vi "only_x_and_y_output.vi"(11 "range":dbl) -> (0 "cycle 2":bool, 1 "range 2":dbl, 2 "Output Y":dbl, 3 "Output X":dbl)   [LabVIEW 2014]
panel:
  out "cycle":bool
  in  "GPIB In":refnum<visa-resource-name>="GPIB0::8::INSTR"
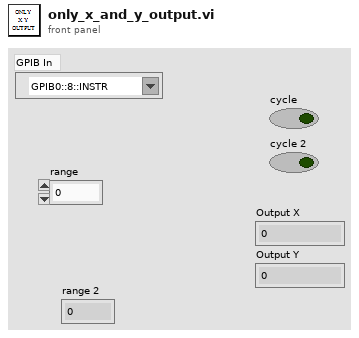
[diagram p1: front panel]
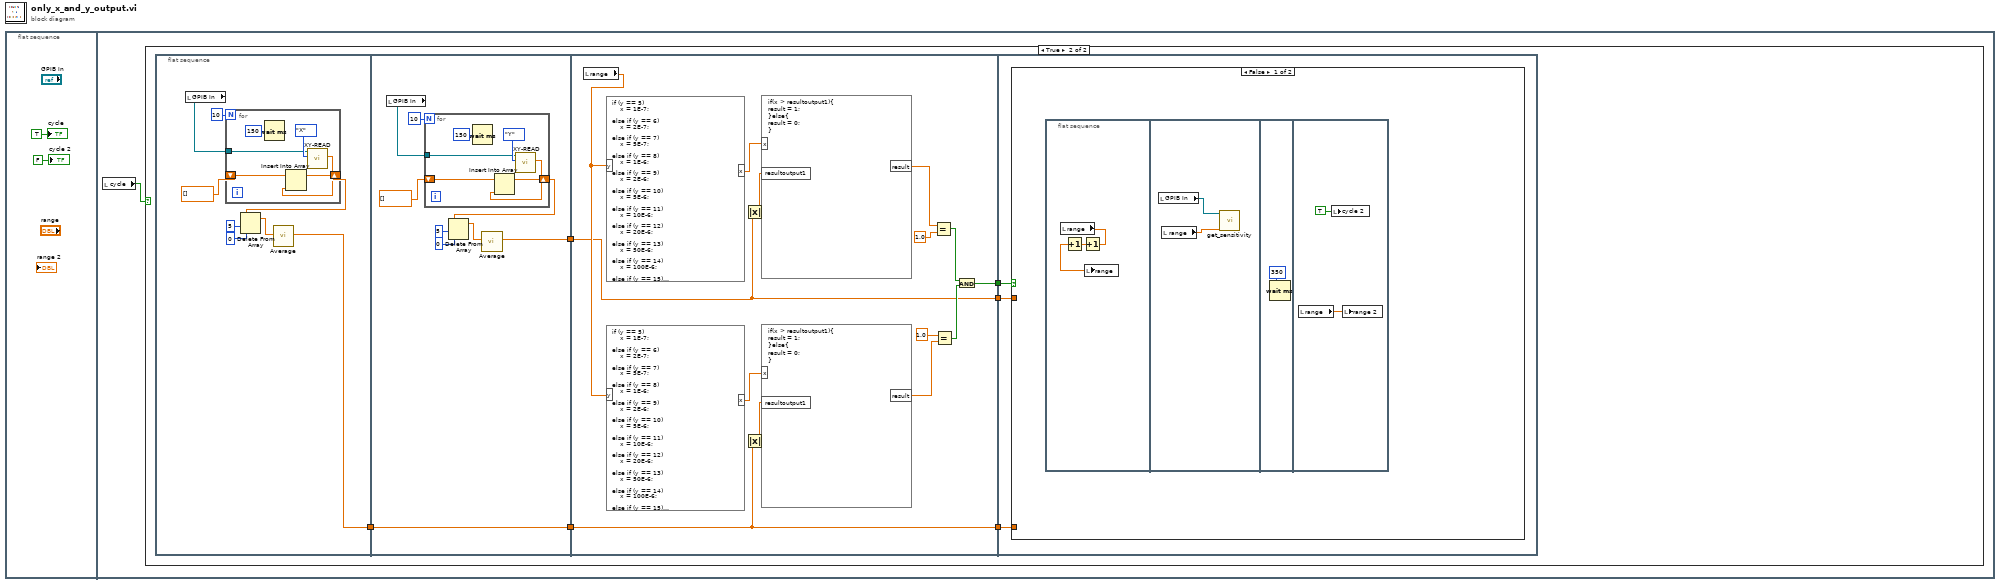
[diagram p0: block diagram]
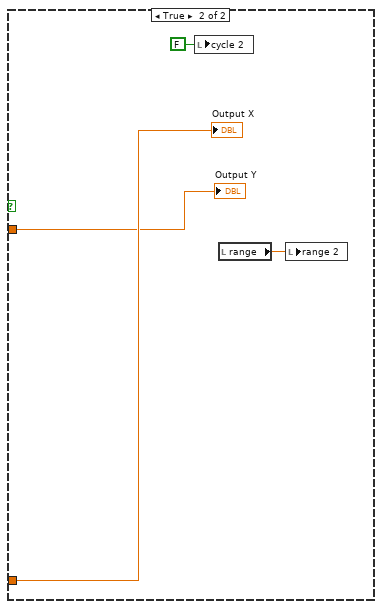
[diagram p3: hidden frame]
diagram:
  n1 = flat-sequence {
    frame #0 {
      "cycle" <- TRUE ("cycle")
      "cycle 2" <- FALSE ("cycle 2")
    }
    frame #1 {
      n2 = local read "cycle"() -> (w3:bool)
      n3 = case shown="True" w3 {
        frame False {
        }
        frame True {
          n4 = flat-sequence {
            tunnel: [w10] -> w7
            tunnel: [w25] -> w9
            tunnel: [w24] -> w8
            tunnel: w7 -> [w24]
            tunnel: w9 -> [w39]
            tunnel: w8 -> [w40]
            tunnel: [w41] -> w6
            tunnel: [w40] -> w5
            tunnel: [w39] -> w4
            tunnel: w6 -> [w55]
            tunnel: w5 -> [w54]
            tunnel: w4 -> [w53]
            frame #0 {
              n5 = local read "GPIB In"() -> (w11:refnum<visa-resource-name>)
              n6 = for {
                N: 10 -> [_]
                tunnel: w11 -> [w22]
                shift-right: [w19] -> w14
                shift-left: dbl[] [] -> [w20]
                n7 = Wait (ms)(milliseconds to wait=u32 150) -> ()  [unwired: 1 out]
                n8 = call "XY-READ.vi"("X/Y ?"=enum16{"X", "Y"}."X" ("Enum"), "SR850 GPIB IN"=w22) -> ("SR850_Reading"=w21:dbl)  [unwired: 7 in, 2 out]
                n9 = Insert Into Array(array=w20, new element=w21) -> (w19:dbl[])  [unwired: 1 in]
              }
              n10 = Delete From Array(array=w14, length=5, index=0) -> (array with subset deleted=w15:dbl[])  [unwired: 1 out]
              n11 = call "Average.vi"("Array"=w15) -> ("Average"=w10:dbl)  [unwired: 9 in, 1 out]
            }
            frame #1 {
              n12 = local read "GPIB In"() -> (w26:refnum<visa-resource-name>)
              n13 = for {
                N: 10 -> [_]
                tunnel: w26 -> [w37]
                shift-right: [w34] -> w29
                shift-left: dbl[] [] -> [w35]
                n14 = Wait (ms)(milliseconds to wait=u32 150) -> ()  [unwired: 1 out]
                n15 = call "XY-READ.vi"("X/Y ?"=enum16{"X", "Y"}."Y" ("Enum"), "SR850 GPIB IN"=w37) -> ("SR850_Reading"=w36:dbl)  [unwired: 7 in, 2 out]
                n16 = Insert Into Array(array=w35, new element=w36) -> (w34:dbl[])  [unwired: 1 in]
              }
              n17 = Delete From Array(array=w29, length=5, index=0) -> (array with subset deleted=w30:dbl[])  [unwired: 1 out]
              n18 = call "Average.vi"("Array"=w30) -> ("Average"=w25:dbl)  [unwired: 9 in, 1 out]
            }
            frame #2 {
              n19 = local read "range"() -> (w48:dbl)
              n20 = formula code="if (y == 5) \n    x = 1E-7;\n\nelse if (y == 6) \n    x = 2E-7;\n\nelse if (y == 7) \n    x = 5E-7;\n\nelse if (y == 8) \n    x = 1E-6;\n\nelse if (y == 9) \n    x = 2E-6;\n\nelse if (y == 10) \n    x = 5E-6;\n\nelse if (y == 11) \n    x = 10E-6;\n\nelse if (y == 12) \n    x = 20E-6;\n\nelse if (y == 13) \n    x = 50E-6;\n\nelse if (y == 14) \n    x = 100E-6;\n\nelse if (y == 15) \n    x = 200E-6;\n\nelse if (y == 16) \n    x = 500E-6;\n\nelse if (y == 17) \n    x = 1E-3;\n\nelse if (y == 18) \n    x = 2E-3;\n\nelse if (y == 19) \n    x = 5E-3;\n\nelse if (y == 20) \n    x = 10E-3;\n\nelse if (y == 21) \n    x = 20E-3;\n\nelse if (y == 22) \n    x = 50E-3;\n\nelse if (y == 23) \n    x = 100E-3;\n\nelse if (y == 24) \n    x = 200E-3;\n\nelse if (y == 25) \n    x = 500E-3;\n\nelse if (y == 26) \n    x = 1;\n\nelse \n    x = 1;"("y"=w48) -> ("x"=w52:dbl)
              n21 = formula code="if (y == 5) \n    x = 1E-7;\n\nelse if (y == 6) \n    x = 2E-7;\n\nelse if (y == 7) \n    x = 5E-7;\n\nelse if (y == 8) \n    x = 1E-6;\n\nelse if (y == 9) \n    x = 2E-6;\n\nelse if (y == 10) \n    x = 5E-6;\n\nelse if (y == 11) \n    x = 10E-6;\n\nelse if (y == 12) \n    x = 20E-6;\n\nelse if (y == 13) \n    x = 50E-6;\n\nelse if (y == 14) \n    x = 100E-6;\n\nelse if (y == 15) \n    x = 200E-6;\n\nelse if (y == 16) \n    x = 500E-6;\n\nelse if (y == 17) \n    x = 1E-3;\n\nelse if (y == 18) \n    x = 2E-3;\n\nelse if (y == 19) \n    x = 5E-3;\n\nelse if (y == 20) \n    x = 10E-3;\n\nelse if (y == 21) \n    x = 20E-3;\n\nelse if (y == 22) \n    x = 50E-3;\n\nelse if (y == 23) \n    x = 100E-3;\n\nelse if (y == 24) \n    x = 200E-3;\n\nelse if (y == 25) \n    x = 500E-3;\n\nelse if (y == 26) \n    x = 1;\n\nelse \n    x = 1;"("y"=w48) -> ("x"=w49:dbl)
              n22 = Absolute Value(x=w39) -> (abs(x)=w51:dbl)
              n23 = Absolute Value(x=w40) -> (abs(x)=w50:dbl)
              n24 = formula code="if(x > resultoutput1){\nresult = 1;\n}else{\nresult = 0;\n}"("x"=w52, "resultoutput1"=w51) -> ("result"=w44:dbl)
              n25 = formula code="if(x > resultoutput1){\nresult = 1;\n}else{\nresult = 0;\n}"("x"=w49, "resultoutput1"=w50) -> ("result"=w46:dbl)
              n26 = Equal?(x=w44, y=1.0 ("x")) -> (x = y?=w43:bool)
              n27 = Equal?(x=1.0, y=w46) -> (x = y?=w42:bool)
              n28 = And(x=w43, y=w42) -> (x .and. y?=w41:bool)
            }
            frame #3 {
              n29 = case shown="False" w55 {
                tunnel: w54 -> [_ w66]
                tunnel: w53 -> [_ w65]
                frame False {
                  n30 = flat-sequence {
                    frame #0 {
                      n31 = local read "range"() -> (w58:dbl)
                      n32 = Increment(x=w58) -> (x+1=w57:dbl)
                      n33 = Increment(x=w57) -> (x+1=w56:dbl)
                      n34 = local write "range"(w56) -> ()
                    }
                    frame #1 {
                      n35 = local read "GPIB In"() -> (w60:refnum<visa-resource-name>)
                      n36 = local read "range"() -> (w59:dbl)
                      n37 = call "get_sensitivity.vi"("input 1"=w59, "SR850 GPIB In"=w60) -> ()  [unwired: 8 in, 2 out]
                    }
                    frame #2 {
                      n38 = Wait (ms)(milliseconds to wait=u32 350) -> ()  [unwired: 1 out]
                    }
                    frame #3 {
                      n39 = local read "range"() -> (w62:dbl)
                      n40 = local write "cycle 2"(TRUE ("cycle 2")) -> ()
                      n41 = local write "range 2"(w62) -> ()
                    }
                  }
                }
                frame True {
                  n42 = local write "cycle 2"(FALSE ("cycle 2")) -> ()
                  n43 = local read "range"() -> (w64:dbl)
                  n44 = local write "range 2"(w64) -> ()
                  "Output Y" <- w65
                  "Output X" <- w66
                }
              }
            }
          }
        }
      }
    }
  }
